vi "CheckIAmEngine.vi"(8 "error in (no error)":errorcluster, 11 "IAmEngine In":refnum<class "IAmEngine.lvclass">) -> (0 "error out":errorcluster, 3 "IAmEngine Out":refnum<class "IAmEngine.lvclass">)   [LabVIEW 2024, in "GLF.lvlib" / "DVRHandler.lvlib"]
uses:
  DVRHandler.lvlib
  IAmEngine/IAmEngine.lvclass
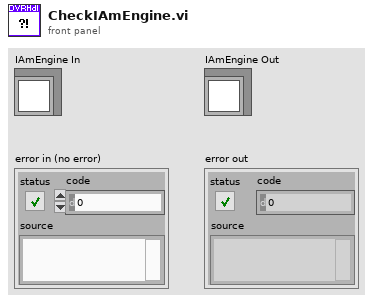
[diagram p1: front panel]
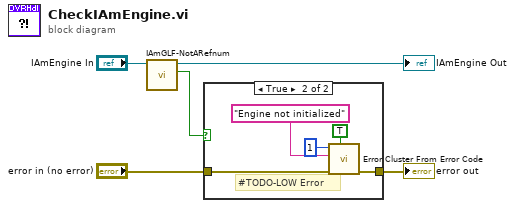
[diagram p0: block diagram]
diagram:
  n1 = call-dynamic "IAmGLF-NotARefnum.vi"("IAmGLF in"="IAmEngine In") -> ("Not A Valid Refnum?"=w1:bool, "IAmGLF out"=→"IAmEngine Out":refnum<class "IAmEngine.lvclass">)  [unwired: 9 in]
  n2 = case shown="True" w1 {
    tunnel: "error in (no error)" -> [w6 w11]
    tunnel: [w6 w10] -> w2
    frame False {
    }
    frame True {
      # "#TODO-LOW Error"
      n3 = call <vilib>:"Error Cluster From Error Code.vi"("show call chain? (False)"=TRUE, "error in (no error)"=w11, "error message (\"\")"="Engine not initialized" ("error message (\"\")"), "error code (0)"=1) -> ("error out"=w10:errorcluster)  [unwired: 5 in]
    }
  }
  "error out" <- w2
